vi "Write MSG Event.vi"(8 "error in (no error)":errorcluster, 10 "MSG Event":refnum<user-event>, 11 "SEQ in":refnum<class "SEQ.lvclass">) -> (0 "error out":errorcluster, 3 "SEQ out":refnum<class "SEQ.lvclass">)   [LabVIEW 2014]
uses:
  SEQ.lvclass
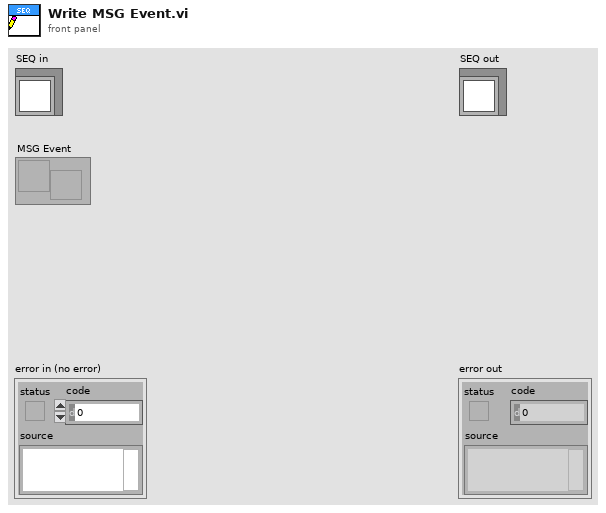
[diagram p1: front panel]
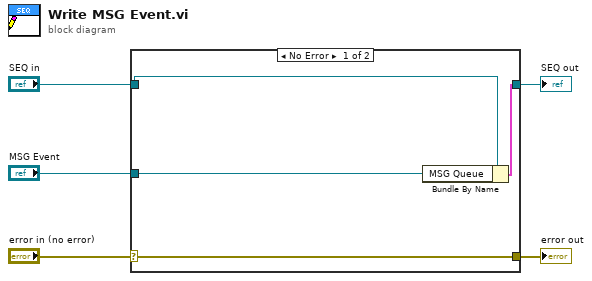
[diagram p0: block diagram]
diagram:
  n1 = case shown="No Error" "error in (no error)" {
    selector: "error in (no error)" -> [w9 w10]
    tunnel: [w9 w10] -> w4
    tunnel: [w7 w11] -> w2
    tunnel: "SEQ in" -> [w8 w11]
    tunnel: "MSG Event" -> [w6 _]
    frame No Error {
      n2 = Bundle By Name(cluster=w8, "MSG Queue"=w6) -> (w7:cluster{})
    }
    frame Error {
    }
  }
  "error out" <- w4
  "SEQ out" <- w2
